vi "Test3v7.vi"() -> ()   [LabVIEW 2013]
uses:
  <vilib>/NI/Tools/String/Tools_String.lvlib
panel:
  out "Length":i32
  out "token array":string[](array[string])
  out "data string":string
  in  "u8 Data[]":u8[](array[numeric]) format="%.0x"
  out "subarray":u8[](array[numeric])
  out "string":string
  out "unsigned byte array":u8[](array[numeric])
  out "index":i32
  out "*(type *) &x":string
  out "size(s)":i32
  out "hex integer string":string[](array[string])
  in  "error in":errorcluster
  out "error out":errorcluster
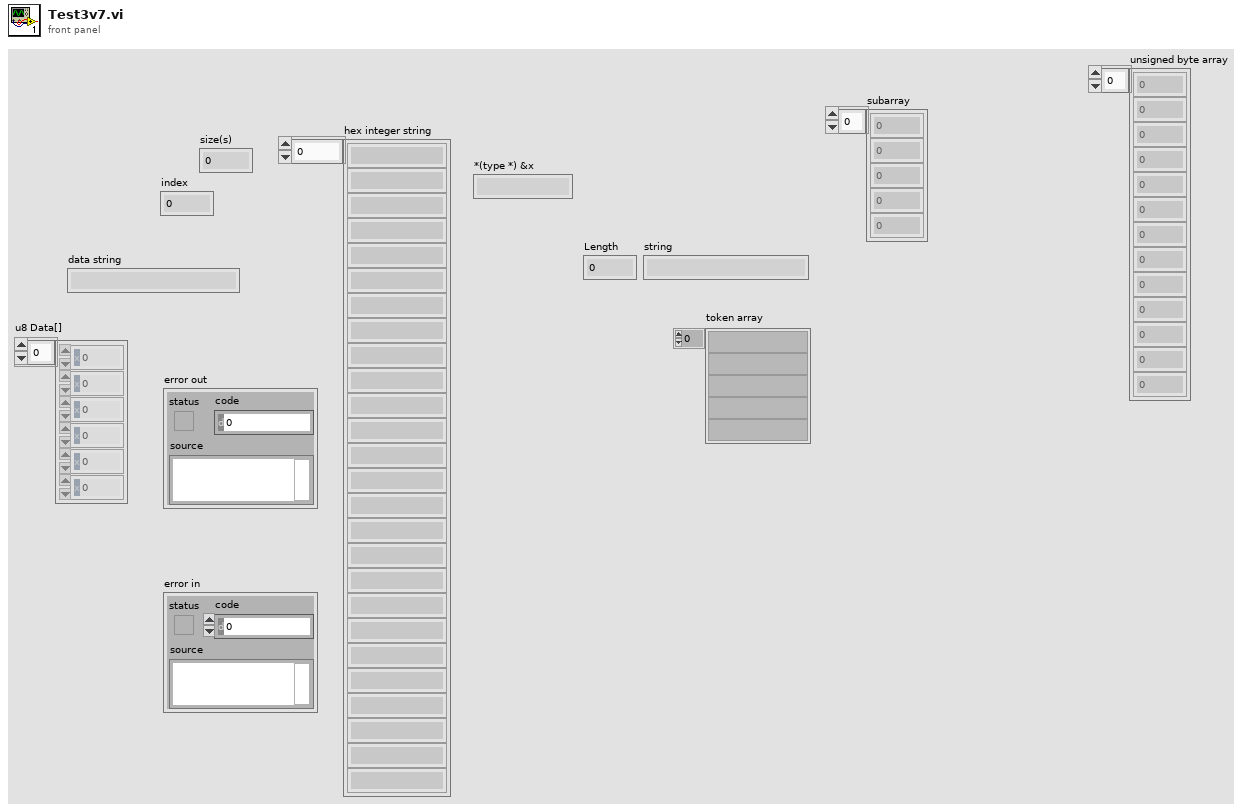
[diagram p1: front panel]
types:
  T1 = enum16{"big-endian, network order", "native, host order", "little-endian"}
  T2 = enum16{"open", "replace", "create", "open or create", "replace or create", "replace or create with confirmation"}
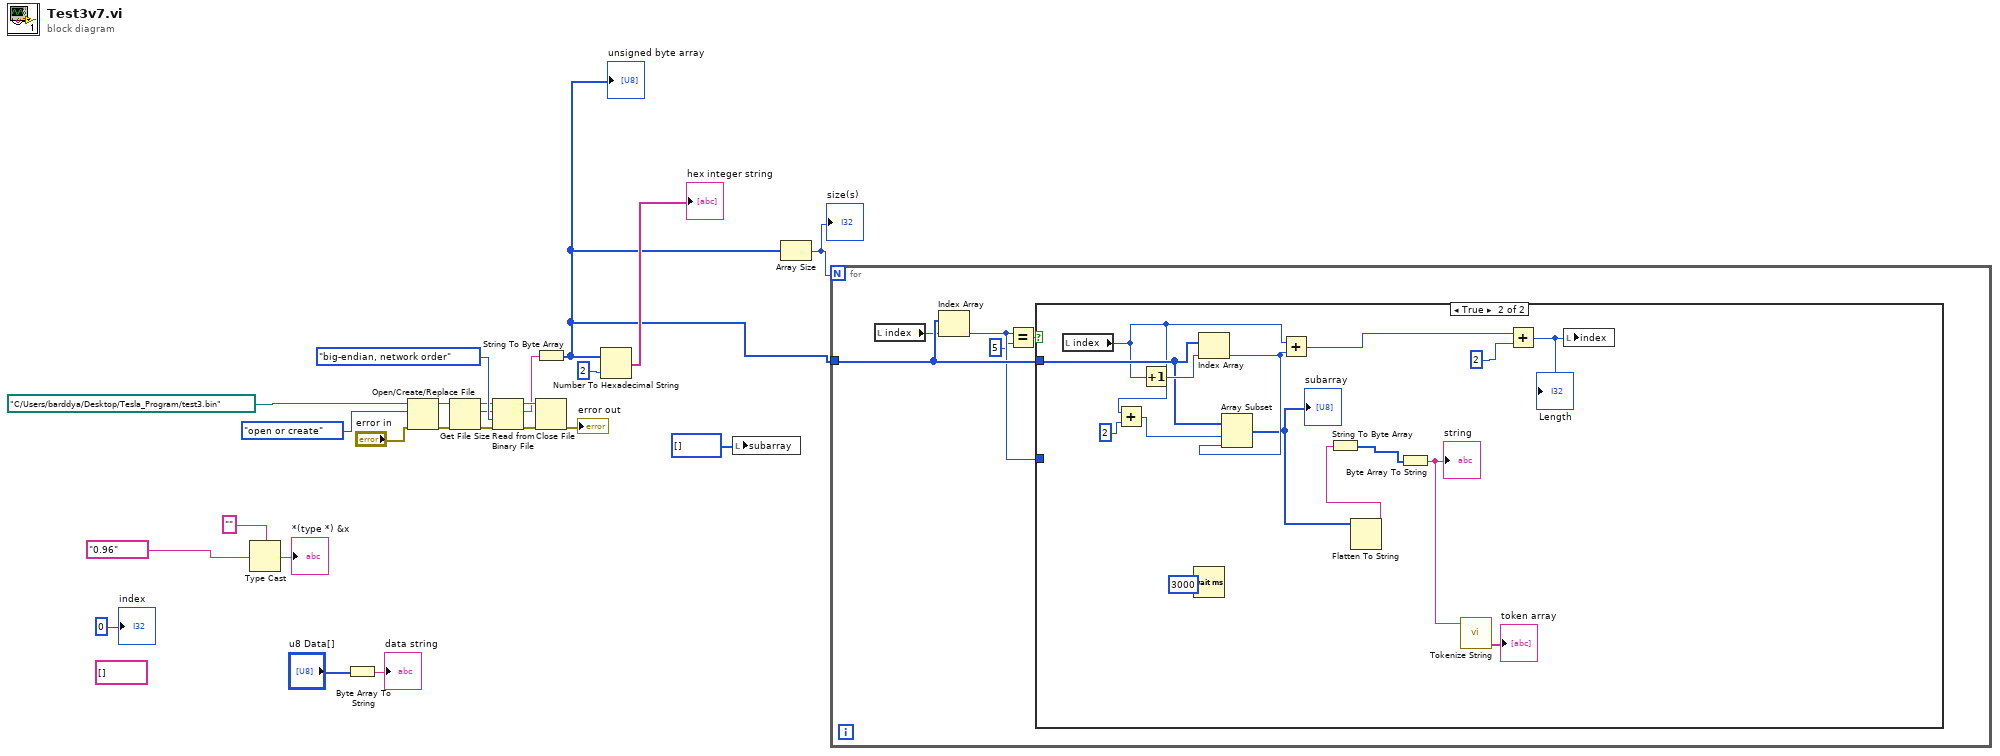
[diagram p0: block diagram]
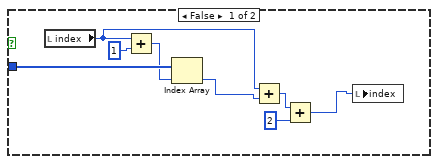
[diagram p2: hidden frame]
diagram:
  (unwired) string[] [] ("subarray")
  n1 = Type Cast(type="", x="0.96") -> (*(type *) &x=→"*(type *) &x":string)
  n2 = Byte Array To String(unsigned byte array="u8 Data[]") -> (string=→"data string":string)
  n3 = Open/Create/Replace File(file path (use dialog)=path "C:/Users/barddya/Desktop/Tesla_Program/test3.bin", error in="error in", operation (0:open)=T2."open or create") -> (refnum out=w17:refnum<file>, error out=w15:errorcluster)  [unwired: 3 in, 1 out]
  n4 = Get File Size(file=w17, error in=w15) -> (refnum out=w16:refnum<file>, size (in bytes)=w13:i64, 0:w14:errorcluster)
  n5 = Read from Binary File(8:w14, 9:T1."big-endian, network order" ("byte order (0:big-endian, network order)"), 10:w13, 11:w16) -> (0:w20:errorcluster, 2:w2:string, 3:w18:refnum<file>)  [unwired: 2 in, 1 out]
  n6 = String To Byte Array(string=w2) -> (unsigned byte array=w1:u8[])
  "unsigned byte array" <- w1
  n7 = Close File(refnum=w18, error in=w20) -> (error out=→"error out":errorcluster)  [unwired: 1 out]
  n8 = Number To Hexadecimal String(1:2, 2:w1) -> (0:→"hex integer string":string[])
  n9 = local write "subarray"(i32[] [] ("subarray")) -> ()
  n10 = Array Size(array=w1) -> (size(s)=w8:i32)
  "size(s)" <- w8
  n11 = for {
    N: w8 -> [_]
    tunnel: w1 -> [w28]
    n12 = local read "index"() -> (w26:i32)
    n13 = Index Array(array=w28, index=w26) -> (element=w27:u8)
    n14 = Equal?(x=w27, y=5) -> (x = y?=w29:bool)
    n15 = case shown="True" w29 {
      tunnel: w28 -> [w37 w50]
      tunnel: w27 -> [_ _]
      frame False {
        n16 = local read "index"() -> (w34:i32)
        n17 = Add(x=w34, y=1) -> (x+y=w35:i32)
        n18 = Index Array(array=w37, index=w35) -> (element=w30:u8)
        n19 = Add(x=w34, y=w30) -> (x+y=w33:i32)
        n20 = Add(x=w33, y=2) -> (x+y=w31:i32)
        n21 = local write "index"(w31) -> ()
      }
      frame True {
        n22 = local read "index"() -> (w48:i32)
        n23 = Add(x=w48, y=2) -> (x+y=w46:i32)
        n24 = Increment(x=w48) -> (x+1=w52:i32)
        n25 = Wait (ms)(milliseconds to wait=3000) -> ()  [unwired: 1 out]
        n26 = Index Array(array=w50, index=w52) -> (element=w43:u8)
        n27 = Array Subset(array=w50, index=w46, length=w43) -> (w41:u8[])
        "subarray" <- w41
        n28 = Add(x=w48, y=w43) -> (x+y=w49:i32)
        n29 = Flatten To String(anything=w41) -> (data string=w40:string)  [unwired: 3 in, 2 out]
        n30 = String To Byte Array(string=w40) -> (unsigned byte array=w44:u8[])
        n31 = Byte Array To String(unsigned byte array=w44) -> (string=w39:string)
        "string" <- w39
        n32 = call <vilib>:"Tokenize String.vi"("input string"=w39) -> ("token array"=→"token array":string[])  [unwired: 3 in, 1 out]
        n33 = Add(x=w49, y=2) -> (x+y=w45:i32)
        "Length" <- w45
        n34 = local write "index"(w45) -> ()
      }
    }
  }
  "index" <- 0
